vi "PH_BeamlineController.set GUI Refs.vi"(0 "Ref in":refnum<vi>, 2 "Class":string, 3 "Beamline Controller GUI Refs":T13={"Sources"=[], "Side Targets"=[], "Targets"=[], "Experiment_VacuumControl_Experiment"=refnum, "special GUI Refs"={"PA-Backreflection-Meas"=refnum, "fs_Synchrolock_Watch"=refnum}, "Beamline Information GUI Refs"={"BL Elements"=[], "Powermeters"={"ns FE"={"GUI Ref"=refnum, "Value"=-1.0}, "fs FE"={"GUI Ref"=refnum, "Value"=-1.0}, "PA"={"GUI Ref"=refnum, "Value"=-1.0}, "MA"={"GUI Ref"=refnum, "Value"=-1.0}, "Z6 green"={"GUI Ref"=refnum, "Value"=-1.0}, "Z6 IR"={"GUI Ref"=refnum, "Value"=-1.0}, "Z6 COS"={"GUI Ref"=refnum, "Value"=-1.0}}, "Efficiency GUI Refs"={"PA Gain"={"GUI Ref"=refnum, "Value"=-1.0}, "MA Gain"={"GUI Ref"=refnum, "Value"=-1.0}, "Z6 green Conversion"={"GUI Ref"=refnum, "Value"=-1.0}, "Z6 Comp Losses"={"GUI Ref"=refnum, "Value"=-1.0}}, "Head GUI Refs"={"PA - 19 - 1"={"in Use"=refnum, "voltage"=refnum}, "PA - 19 - 2"={"in Use"=refnum, "voltage"=refnum}, "PA - 45"={"in Use"=refnum, "voltage"=refnum}, "PA - 45 - DP"={"in Use"=refnum, "voltage"=refnum}, "MA - 1"={"in Use"=refnum, "voltage"=refnum}, "MA - 2"={"in Use"=refnum, "voltage"=refnum}, "MA - 3"={"in Use"=refnum, "voltage"=refnum}, "MA - 4"={"in Use"=refnum, "voltage"=refnum}, "MA - 5"={"in Use"=refnum, "voltage"=refnum}, "MA - FR"={"in Use"=refnum, "voltage"=refnum}}, "System Information GUI Refs"={"Laser"=refnum, "PreAmp"=refnum, "MainAmp"=refnum, "Emergency Off"=refnum, "Exp 1"=refnum, "Exp 2"=refnum, "Exp 3"=refnum, "Exp 4"=refnum, "Timing Mode GUI Ref"=refnum}}}, 5 "error in":errorcluster) -> (14 "Ref out":refnum<vi>, 19 "error out":errorcluster)   [LabVIEW 2014, in "PH_BeamlineController.lvlib"]
uses:
  PH_BeamlineController.lvlib
  PH_BeamlineController.Source Attributes.ctl
  PH_BeamlineController.Sources.ctl
  PH_BeamlineController.PA DP Target Attributes.ctl
  PH_BeamlineController.PA DP Targets.ctl
  PH_BeamlineController.Target Attributes.ctl
  PH_BeamlineController.Targets.ctl
  PH_BeamlineController.special GUI Refs.ctl
  PH_BeamlineInformation/PH_BeamlineInformation.GUI Ref.ctl
  PH_Beamline_Chief/PH_Beamline_Chief.Section.ctl
  PH_BeamlineInformation/PH_BeamlineInformation.Powermeter.ctl
  PH_BeamlineInformation/PH_BeamlineInformation.Efficiency.ctl
  PH_Basics/PH_SystemInformation/PH_SystemInformation.GUI Refs.ctl
  PH_BeamlineInformation/PH_BeamlineInformation.lvlib
  PH_Beamline_Chief/PH_Beamline_Chief.lvlib
  PH_Basics/PH_SystemInformation/PH_SystemInformation.lvlib
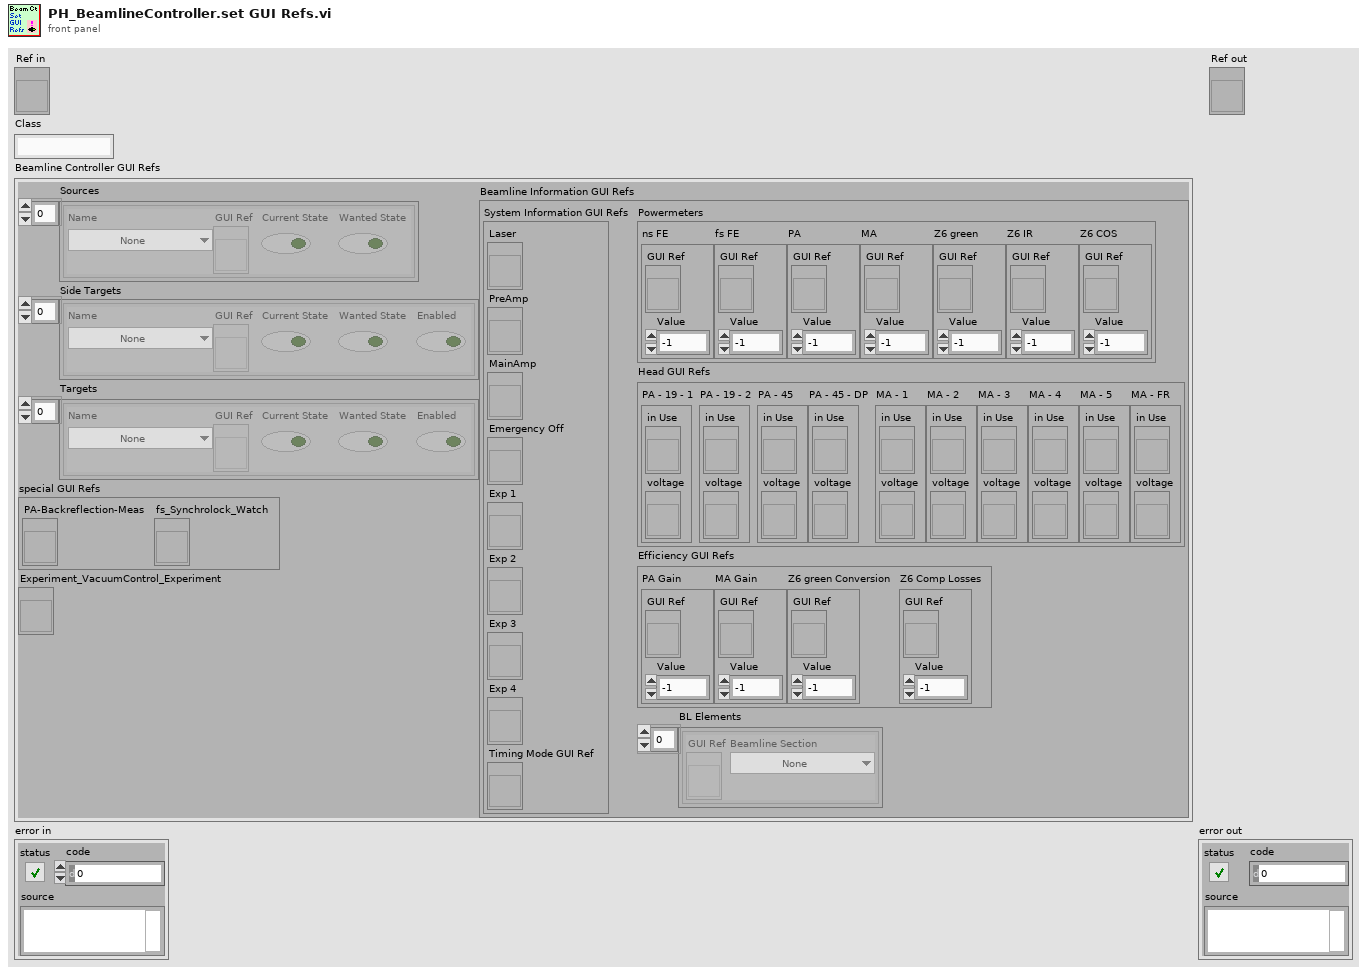
[diagram p1: front panel]
types:
  T1 = typedef "PH_BeamlineController.lvlib/PH_BeamlineController.Source Attributes.ctl" = cluster{"Name":T2, "GUI Ref":refnum<vi>, "Current State":bool, "Wanted State":bool}
  T2 = typedef "PH_BeamlineController.lvlib/PH_BeamlineController.Sources.ctl" = enum16{"None", "YLF", "fs-Frontend", "ns-Frontend", "YLF and ns-Frontend", "fs- and ns-Frontend"}
  T3 = typedef "PH_BeamlineController.lvlib/PH_BeamlineController.PA DP Target Attributes.ctl" = cluster{"Name":T4, "GUI Ref":refnum<vi>, "Current State":bool, "Wanted State":bool, "Enabled":bool}
  T4 = typedef "PH_BeamlineController.lvlib/PH_BeamlineController.PA DP Targets.ctl" = enum16{"None", "Dump PA Delayed Beam", "Dump PA Undelayed Beam", "Dumps PA Delayed and Undelayed Beam"}
  T5 = typedef "PH_BeamlineController.lvlib/PH_BeamlineController.Target Attributes.ctl" = cluster{"Name":T6, "GUI Ref":refnum<vi>, "Current State":bool, "Wanted State":bool, "Enabled":bool}
  T6 = typedef "PH_BeamlineController.lvlib/PH_BeamlineController.Targets.ctl" = enum16{"None", "PreAmp", "Dump Exp Laserlab", "Exp Laserlab", "Calorimeter", "Dump Exp Laserbay", "Exp Laserbay", "Dump Exp Z6", "Exp Z6"}
  T7 = typedef "PH_BeamlineController.lvlib/PH_BeamlineController.special GUI Refs.ctl" = cluster{"PA-Backreflection-Meas":refnum<vi>, "fs_Synchrolock_Watch":refnum<vi>}
  T8 = typedef "PH_BeamlineInformation.lvlib/PH_BeamlineInformation.GUI Ref.ctl" = cluster{"BL Elements":cluster{"GUI Ref":refnum<vi>, "Beamline Section":T9}[], "Powermeters":T10, "Efficiency GUI Refs":T11, "Head GUI Refs":cluster{"PA - 19 - 1":cluster{"in Use":refnum<vi>, "voltage":refnum<vi>}, "PA - 19 - 2":cluster{"in Use":refnum<vi>, "voltage":refnum<vi>}, "PA - 45":cluster{"in Use":refnum<vi>, "voltage":refnum<vi>}, "PA - 45 - DP":cluster{"in Use":refnum<vi>, "voltage":refnum<vi>}, "MA - 1":cluster{"in Use":refnum<vi>, "voltage":refnum<vi>}, "MA - 2":cluster{"in Use":refnum<vi>, "voltage":refnum<vi>}, "MA - 3":cluster{"in Use":refnum<vi>, "voltage":refnum<vi>}, "MA - 4":cluster{"in Use":refnum<vi>, "voltage":refnum<vi>}, "MA - 5":cluster{"in Use":refnum<vi>, "voltage":refnum<vi>}, "MA - FR":cluster{"in Use":refnum<vi>, "voltage":refnum<vi>}}, "System Information GUI Refs":T12}
  T9 = typedef "PH_Beamline_Chief.lvlib/PH_Beamline_Chief.Section.ctl" = enum16{"None", "YLF", "fs", "fs-YLF", "ns", "PA-Input", "PA-Undelay", "PA-Delay", "PA-before-Bypass", "PA", "PA-Bypass", "PA-Exit", "PA-LL", "LL", "PA-MA", "MA-Exit", "MA-Z6", "Z6", "MA-LB", "LB-TB2", "LB-TB3"}
  T10 = typedef "PH_BeamlineInformation.lvlib/PH_BeamlineInformation.Powermeter.ctl" = cluster{"ns FE":cluster{"GUI Ref":refnum<vi>, "Value":dbl}, "fs FE":cluster{"GUI Ref":refnum<vi>, "Value":dbl}, "PA":cluster{"GUI Ref":refnum<vi>, "Value":dbl}, "MA":cluster{"GUI Ref":refnum<vi>, "Value":dbl}, "Z6 green":cluster{"GUI Ref":refnum<vi>, "Value":dbl}, "Z6 IR":cluster{"GUI Ref":refnum<vi>, "Value":dbl}, "Z6 COS":cluster{"GUI Ref":refnum<vi>, "Value":dbl}}
  T11 = typedef "PH_BeamlineInformation.lvlib/PH_BeamlineInformation.Efficiency.ctl" = cluster{"PA Gain":cluster{"GUI Ref":refnum<vi>, "Value":dbl}, "MA Gain":cluster{"GUI Ref":refnum<vi>, "Value":dbl}, "Z6 green Conversion":cluster{"GUI Ref":refnum<vi>, "Value":dbl}, "Z6 Comp Losses":cluster{"GUI Ref":refnum<vi>, "Value":dbl}}
  T12 = typedef "PH_SystemInformation.lvlib/PH_SystemInformation.GUI Refs.ctl" = cluster{"Laser":refnum<vi>, "PreAmp":refnum<vi>, "MainAmp":refnum<vi>, "Emergency Off":refnum<vi>, "Exp 1":refnum<vi>, "Exp 2":refnum<vi>, "Exp 3":refnum<vi>, "Exp 4":refnum<vi>, "Timing Mode GUI Ref":refnum<vi>}
  T13 = cluster{"Sources":T1[], "Side Targets":T3[], "Targets":T5[], "Experiment_VacuumControl_Experiment":refnum<vi>, "special GUI Refs":T7, "Beamline Information GUI Refs":T8}
  T14 = typedef "PH_BeamlineController.lvlib/PH_BeamlineController.i attribute.ctl" = cluster{"Vacuum Exp LB":cluster{"Channel":string, "Limit [mbar]":dbl, "Pressure [mbar]":dbl, "GUI Ref":refnum<vi>}, "Sources":T1[], "PA DP Targets":T3[], "Path":cluster{"Source":T2, "PA DP Target":T4, "Target":T6}, "Targets":cluster{"Name":T6, "GUI Ref":refnum<vi>, "Current State":bool, "Wanted State":bool, "Enabled":bool}[], "Status Tags":cluster{"Name":string, "Status":T15}[], "special GUI Refs":T7}
  T15 = typedef "PH_StatusHandler.lvlib/PH_StatusHandler.Status.ctl" = i16
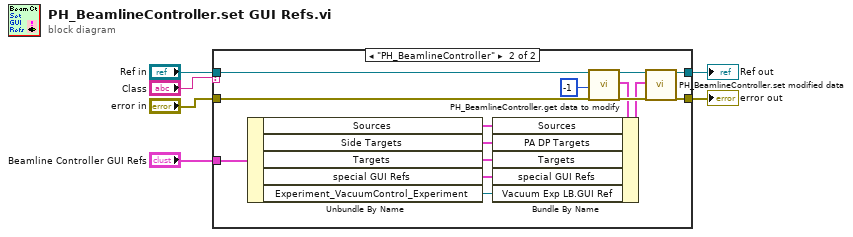
[diagram p0: block diagram]
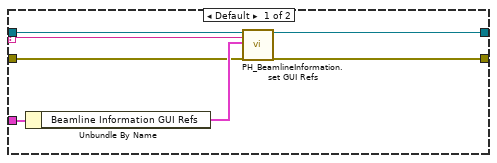
[diagram p2: hidden frame]
diagram:
  n1 = case shown="\"PH_BeamlineController\"" "Class" {
    selector: "Class" -> [w12 _]
    tunnel: "Ref in" -> [w13 w23]
    tunnel: "error in" -> [w9 w22]
    tunnel: [w7 w15] -> w4
    tunnel: [w8 w14] -> w3
    tunnel: "Beamline Controller GUI Refs" -> [w11 w21]
    frame Default {
      n2 = Unbundle By Name(w11) -> ("Beamline Information GUI Refs"=w10:T8)
      n3 = call "PH_BeamlineInformation.set GUI Refs.vi"("Ref in"=w13, "Class"=w12, "BeamlineInformation GUI Refs"=w10, "error in"=w9) -> ("Ref out"=w7:refnum<vi>, "error out"=w8:errorcluster)  [unwired: 14 in]
    }
    frame "PH_BeamlineController" {
      n4 = Unbundle By Name(w21) -> ("Sources"=w20:T1[], "Side Targets"=w18:T3[], "Targets"=w19:T5[], "special GUI Refs"=w17:T7, "Experiment_VacuumControl_Experiment"=w16:refnum<vi>)
      n5 = call "PH_BeamlineController.get data to modify.vi"("i ref in"=w23, "ms timeout (10000)"=-1, "error in (no error)"=w22) -> ("i ref out"=w26:refnum<vi>, "i attribute"=w24:T14, "error out"=w28:errorcluster)  [unwired: 13 in, 1 out]
      n6 = Bundle By Name(cluster=w24, "Sources"=w20, "PA DP Targets"=w18, "Targets"=w19, "special GUI Refs"=w17, "Vacuum Exp LB.GUI Ref"=w16) -> (w25:T14)
      n7 = call "PH_BeamlineController.set modified data.vi"("i ref in"=w26, "i attribute"=w25, "error in (no error)"=w28) -> ("i ref out"=w15:refnum<vi>, "error out"=w14:errorcluster)  [unwired: 15 in]
    }
  }
  "error out" <- w3
  "Ref out" <- w4
